vi "ConfigureCamera.vi"(6 "Line name":string="Line 0", 8 "error in (no error)":errorcluster, 9 "Frames Per Second":dbl, 10 "Automatic frame rate":string, 11 "Refnum in":T1) -> (0 "error out":errorcluster, 3 "Refnum out":T1)   [LabVIEW 2017]
doc: "Configure camera for acquiring. This will throw an error for non USB3 video compliant cameras.s"
uses:
  <vilib>/userdefined/High Color/IMAQdx.ctl
  <resource>/objmgr/imaqdx.rc
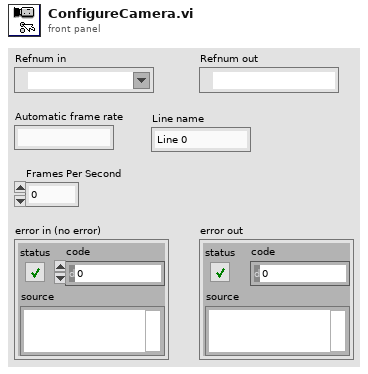
[diagram p1: front panel]
types:
  T1 = typedef "IMAQdx.ctl" = refnum<k21>
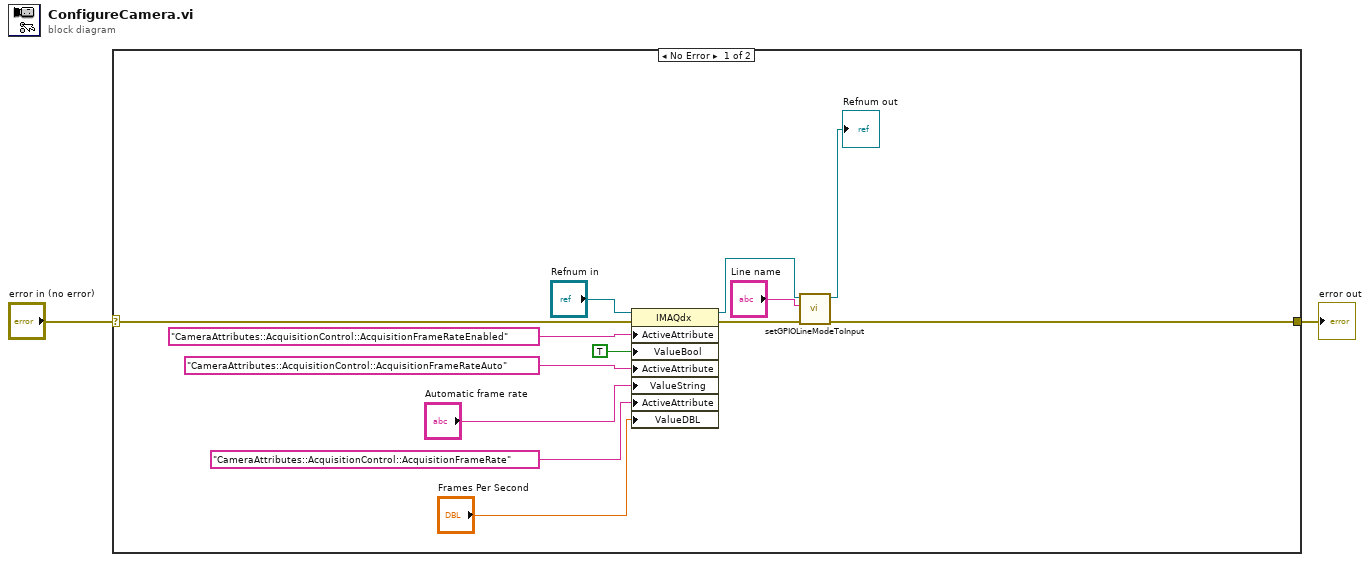
[diagram p0: block diagram]
diagram:
  n1 = case shown="No Error" "error in (no error)" {
    selector: "error in (no error)" -> [w4 w16]
    tunnel: [w3 w16] -> w2
    frame No Error {
      n2 = property class="IMAQdx"(reference="Refnum in", error in=w4, "ActiveAttribute"="CameraAttributes::AcquisitionControl::AcquisitionFrameRateEnabled", "ValueBool"=TRUE, "ActiveAttribute"="CameraAttributes::AcquisitionControl::AcquisitionFrameRateAuto", "ValueString"="Automatic frame rate", "ActiveAttribute"="CameraAttributes::AcquisitionControl::AcquisitionFrameRate", "ValueDBL"="Frames Per Second") -> (reference out=w7:T1, error out=w5:errorcluster)
      n3 = call "setGPIOLineModeToInput.vi"("error in (no error)"=w5, "GPIO line"="Line name", "IMAQdx Session in"=w7) -> ("error out"=w3:errorcluster, "IMAQdx Session out"=→"Refnum out":T1)  [unwired: 7 in]
    }
    frame Error {
    }
  }
  "error out" <- w2
